vi "R45_1-RT.vi"() -> ()   [LabVIEW 2016]
uses:
  <vilib>/rvi/interface/nirviOpenFPGA/nirviOpenFPGA.xnode
  <vilib>/rvi/interface/nirviReadWriteControl/nirviReadWriteControl.xnode
  Common-Control/Beamline sections/R45/R45_1/R45_1-FPGA.vi
  <vilib>/rvi/errors/niLvFpgaAdjustHostInterfaceError.vi
  <vilib>/Utility/error.llb/Error Cluster From Error Code.vi
  NiFpgaLv.dll
  Glassman Control.ctl
  GP307 cluster.ctl
  Controls/GV states.ctl
  Controls/Faraday cup states.ctl
  Controls/Aperture states.ctl
  Cryo Readback.ctl
  <vilib>/NI_Real-Time Target Support.lvlib
  FPGA Bitfiles/PRIMEControl2017_FPGATarget10_R45-1-FPGA_JlC5-fMslM8.lvbitx
  <vilib>/FPGAPlugInAG/cRIO-9067/niLvFpga_Open_cRIO-9067.vi
panel:
  in  "Tab Control":T1(tab)
  out "Left-Steerer voltage set":dbl
  out "Left-Steerer HV Enable":bool
  out "Right-Steerer HV Enable":bool
  out "Right-Steerer voltage set":dbl
  out "Up-Steerer Voltage Set":dbl
  out "Up-Steerer HV Enable":bool
  out "Down-Steerer HV Enable":bool
  out "Down-Steerer Voltage Set":dbl
  out "Up Steerer readback.I-monitor":fxp<+/-,26,5>
  out "Up Steerer readback.V-monitor":fxp<+/-,26,7>
  out "Down Steerer readback.I-monitor":fxp<+/-,26,5>
  out "Down Steerer readback.V-monitor":fxp<+/-,26,7>
  out "Left Steerer readback.I-monitor":fxp<+/-,26,5>
  out "Left Steerer readback.V-monitor":fxp<+/-,26,7>
  out "Right Steerer readback.I-monitor":fxp<+/-,26,5>
  out "Right Steerer readback.V-monitor":fxp<+/-,26,7>
  out "Cryo status":u8[](array[numeric])
  out "Cryo On-time":u8[](array[numeric])
  out "Cryo 1st stage temp":u8[](array[numeric])
  out "2nd stage temp":u8[](array[numeric])
  out "Time since repurge":u8[](array[numeric])
  out "Vac cluster 2 Interlock":bool
  out "Vac cluster 2 Interlock bypass":bool
  out "Vac cluster 1 interlock bypass":bool
  out "Status":string
  out "On-time":string
  out "1st Stage Temp":string
  out "2nd Stage Temp":string
  out "Time since re-purge":string
  out "Cryo Readback":T2
  out "Vac Cluster 1 Ion Gauge 1":u8[](array[numeric])
  out "Vac Cluster 1 Convectron 1":u8[](array[numeric])
  out "Switch Image Convectron 1":dbl
  out "Switch Image Vac Cluster":T3
  out "Switch Image Ion Gauge 1":dbl
  out "Vac Cluster 1 Ion Gauge 2":u8[](array[numeric])
  out "Vac Cluster 1 Convectron 2":u8[](array[numeric])
  out "Cryo Pump GV status 2":T4
  out "Cryo Pump GV status":T5
  out "Beamline GV 1 status 2":T4
  out "Beamline GV 1 status":T5
  out "Switch Image FC Position":cluster{"IN sensor":bool, "OUT sensor":bool}
  out "Switch Image Aperture Position":cluster{"IN sensor":bool, "OUT sensor":bool}
  out "Aperture Status":T6
  out "FC Status":T7
  out "Cryo Pump GV Actuator":bool
  out "Switch Mag Aperture actuator":bool
  out "Switch Mag FC actuator":bool
  out "Beamline GV 1 Actuator":bool
  out "Error Reporter":errorcluster
  out "Interlock loop error":errorcluster
  out "Actuator-Sensor Loop error":errorcluster
  out "Cryo loop error":errorcluster
  out "Vac cluster loop error":errorcluster
  out "HV readback loop error":errorcluster
  out "HV control loop error":errorcluster
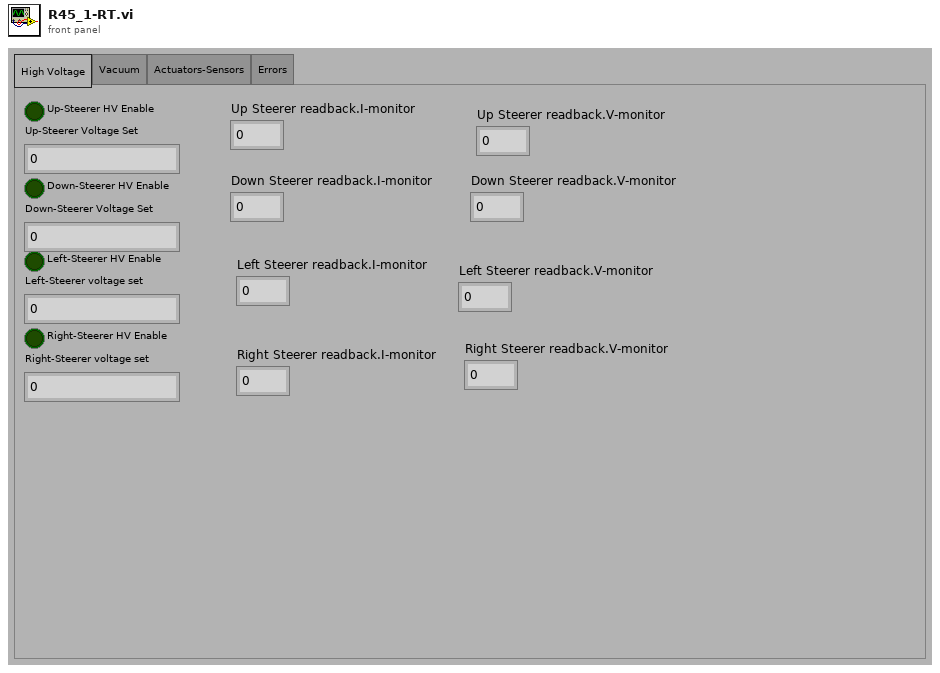
[diagram p1: front panel]
types:
  T1 = enum32{"High Voltage", "Vacuum", "Actuators-Sensors", "Errors"}
  T2 = typedef "Cryo Readback.ctl" = cluster{"Status":string, "On-time":string, "1st Stage Temp":string, "2nd Stage Temp":string, "Time since re-purge":string}
  T3 = typedef "GP307 cluster.ctl" = cluster{"Ion gauge 1":string, "Convectron  Gauge 1 ":string, "Ion Gauge 2":string, "Convectrom Gauge 2":string}
  T4 = cluster{"OPEN sensor":bool, "Closed sensor":bool}
  T5 = typedef "GV states.ctl" = enum16{"status unclear", "closed", "open"}
  T6 = typedef "Aperture states.ctl" = enum16{"Aperture status unclear", "Aperture in", "Aperture out"}
  T7 = typedef "Faraday cup states.ctl" = enum16{"FC status unclear", "FC in", "FC out"}
  T8 = typedef "Glassman Control.ctl" = cluster{"V-program":fxp<+/-,16,5>, "HV Enable":bool}
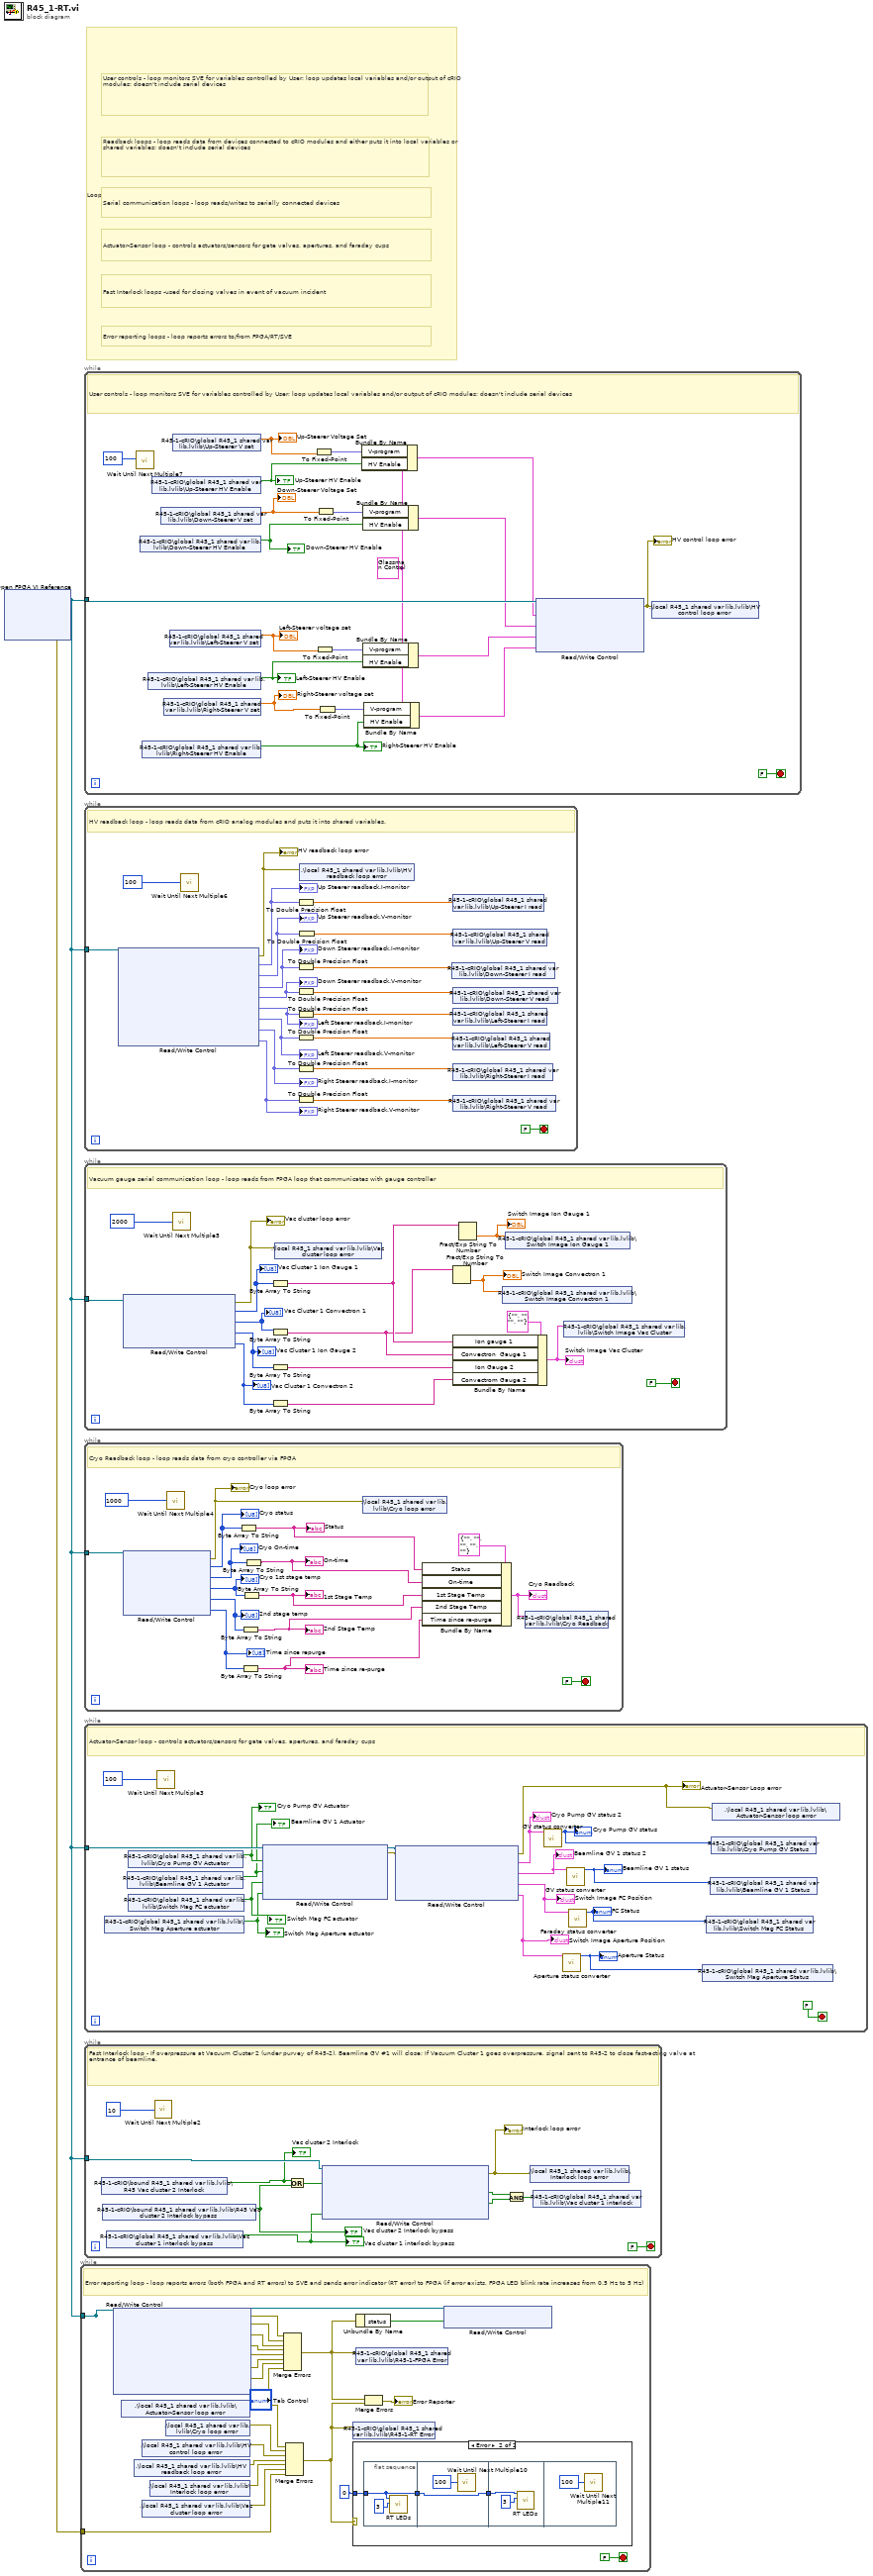
[diagram p0: block diagram]
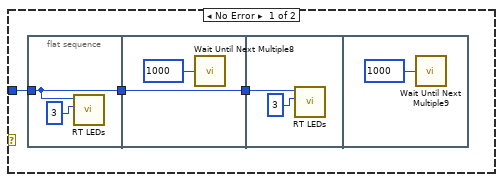
[diagram p2: hidden frame]
diagram:
  # "Actuator-Sensor loop - controls actuators/sensors for gate valves, apertures, and faraday cups"
  # "Fast Interlock loops -used for closing valves in event of vacuum incident"
  # "Error reporting loops - loop reports errors to/from FPGA/RT/SVE"
  # "Serial communication loops - loop reads/writes to serially connected devices"
  # "Readback loops - loop reads data from devices connected to cRIO modules and either puts it into local variables or shared variables; doesn't include serial devices"
  # "User controls - loop monitors SVE for variables controlled by User; loop updates local variables and/or output of cRIO modules; doesn't include serial devices"
  # "Loop legend - loops are color coded by responsibility"
  n1 = xnode "Open FPGA VI Reference"() -> ("FPGA VI Reference Out"=w2:refnum<k20>, "error out"=w1:errorcluster)  [unwired: 2 in]
  n2 = while {
    tunnel: [w25] -> _
    tunnel: w2 -> [w25]
    tunnel: w1 -> [w5]
    stop <- FALSE stop-if-true
    # "Error reporting loop - loop reports errors (both FPGA and RT errors) to SVE and sends error indicator (RT error) to FPGA (if error exists, FPGA LED blink rate increases from 0.5 Hz to 5 Hz)"
    n3 = xnode "Read/Write Control"("FPGA VI Reference In"=w25) -> ("FPGA VI Reference Out"=w15:refnum<k20>, "error out"=w24:errorcluster, "Vac and GV interlock error"=w23:errorcluster, "Position-Sensor readback error"=w22:errorcluster, "Cup-Aperture Control Loop Error"=w21:errorcluster, "Cryo pump error"=w20:errorcluster, "HV readback error"=w19:errorcluster, "HV Control error"=w18:errorcluster, "Vacuum Gauge 1 error"=w17:errorcluster)  [unwired: 1 in]
    n4 = shared-variable ".\\local R45_1 shared var lib.lvlib\\Actuator-Sensor loop error"() -> (w11:errorcluster)  [unwired: 1 in, 1 out]
    n5 = shared-variable ".\\local R45_1 shared var lib.lvlib\\HV readback loop error"() -> (w8:errorcluster)  [unwired: 1 in, 1 out]
    n6 = shared-variable ".\\local R45_1 shared var lib.lvlib\\HV control loop error"() -> (w9:errorcluster)  [unwired: 1 in, 1 out]
    n7 = shared-variable ".\\local R45_1 shared var lib.lvlib\\Vac cluster loop error"() -> (w6:errorcluster)  [unwired: 1 in, 1 out]
    n8 = shared-variable ".\\local R45_1 shared var lib.lvlib\\Interlock loop error"() -> (w7:errorcluster)  [unwired: 1 in, 1 out]
    n9 = shared-variable ".\\local R45_1 shared var lib.lvlib\\Cryo loop error"() -> (w10:errorcluster)  [unwired: 1 in, 1 out]
    n10 = Merge Errors(w24, w23, w22, w21, w20, w19, w18, w17) -> (w16:errorcluster)
    n11 = Merge Errors(w11, w10, w9, w8, w7, w6, w5) -> (w3:errorcluster)
    n12 = case shown="Error" w3 {
      tunnel: 0 -> [w28 w36]
      frame No Error {
        n13 = flat-sequence {
          tunnel: w28 -> [w29]
          tunnel: [w29] -> w26
          tunnel: [w31] -> w27
          tunnel: w26 -> [w31]
          tunnel: w27 -> [w33]
          frame #0 {
            n14 = call <vilib>:"RT LEDs.vi"("State"=3, "LED Num"=w29) -> ()  [unwired: 4 in, 2 out]
          }
          frame #1 {
            n15 = call "Wait Until Next Multiple8"("Count(mSec)"=u16 1000) -> ()  [unwired: 1 out]
          }
          frame #2 {
            n16 = call <vilib>:"RT LEDs.vi"("State"=3, "LED Num"=w33) -> ()  [unwired: 4 in, 2 out]
          }
          frame #3 {
            n17 = call "Wait Until Next Multiple9"("Count(mSec)"=u16 1000) -> ()  [unwired: 1 out]
          }
        }
      }
      frame Error {
        n18 = flat-sequence {
          tunnel: [w39] -> w38
          tunnel: w36 -> [w39]
          tunnel: w38 -> [w41]
          tunnel: [w41] -> w37
          tunnel: w37 -> [w43]
          frame #0 {
            n19 = call <vilib>:"RT LEDs.vi"("State"=3, "LED Num"=w39) -> ()  [unwired: 4 in, 2 out]
          }
          frame #1 {
            n20 = call "Wait Until Next Multiple10"("Count(mSec)"=u16 100) -> ()  [unwired: 1 out]
          }
          frame #2 {
            n21 = call <vilib>:"RT LEDs.vi"("State"=3, "LED Num"=w43) -> ()  [unwired: 4 in, 2 out]
          }
          frame #3 {
            n22 = call "Wait Until Next Multiple11"("Count(mSec)"=u16 100) -> ()  [unwired: 1 out]
          }
        }
      }
    }
    n23 = shared-variable "R45-1-cRIO\\global R45_1 shared var lib.lvlib\\R45-1-RT Error"(w3) -> ()  [unwired: 1 in, 1 out]
    n24 = shared-variable "R45-1-cRIO\\global R45_1 shared var lib.lvlib\\R45-1-FPGA Error"(w16) -> ()  [unwired: 1 in, 1 out]
    n25 = Unbundle By Name(w16) -> ("status"=w14:bool)
    n26 = Merge Errors(w16, w3) -> (→"Error Reporter":errorcluster)
    n27 = xnode "Read/Write Control"("FPGA VI Reference In"=w15, "RT error"=w14) -> ()  [unwired: 1 in, 2 out]
  }
  n28 = while {
    tunnel: w2 -> [w66]
    stop <- FALSE stop-if-true
    w55 = T8 {"V-program"=0.0, "HV Enable"=FALSE} ("Glassman Control")
    # "User controls - loop monitors SVE for variables controlled by User; loop updates local variables and/or output of cRIO modules; doesn't include serial devices"
    n29 = call "Wait Until Next Multiple7"("Count(mSec)"=u32 100 ("millisecond multiple")) -> ()  [unwired: 1 out]
    n30 = shared-variable "R45-1-cRIO\\global R45_1 shared var lib.lvlib\\Down-Steerer HV Enable"() -> (w51:bool)  [unwired: 1 in, 1 out]
    "Down-Steerer HV Enable" <- w51
    n31 = shared-variable "R45-1-cRIO\\global R45_1 shared var lib.lvlib\\Right-Steerer HV Enable"() -> (w47:bool)  [unwired: 1 in, 1 out]
    "Right-Steerer HV Enable" <- w47
    n32 = shared-variable "R45-1-cRIO\\global R45_1 shared var lib.lvlib\\Left-Steerer HV Enable"() -> (w49:bool)  [unwired: 1 in, 1 out]
    "Left-Steerer HV Enable" <- w49
    n33 = shared-variable "R45-1-cRIO\\global R45_1 shared var lib.lvlib\\Up-Steerer HV Enable"() -> (w54:bool)  [unwired: 1 in, 1 out]
    "Up-Steerer HV Enable" <- w54
    n34 = shared-variable "R45-1-cRIO\\global R45_1 shared var lib.lvlib\\Down-Steerer V set"() -> (w52:dbl)  [unwired: 1 in, 1 out]
    "Down-Steerer Voltage Set" <- w52
    n35 = shared-variable "R45-1-cRIO\\global R45_1 shared var lib.lvlib\\Right-Steerer V set"() -> (w48:dbl)  [unwired: 1 in, 1 out]
    "Right-Steerer voltage set" <- w48
    n36 = shared-variable "R45-1-cRIO\\global R45_1 shared var lib.lvlib\\Left-Steerer V set"() -> (w50:dbl)  [unwired: 1 in, 1 out]
    "Left-Steerer voltage set" <- w50
    n37 = shared-variable "R45-1-cRIO\\global R45_1 shared var lib.lvlib\\Up-Steerer V set"() -> (w53:dbl)  [unwired: 1 in, 1 out]
    "Up-Steerer Voltage Set" <- w53
    n38 = To Fixed-Point(number=w53) -> (fixed-point=w59:fxp<+/-,20,5>)  [unwired: 1 in]
    n39 = To Fixed-Point(number=w50) -> (fixed-point=w63:fxp<+/-,20,5>)  [unwired: 1 in]
    n40 = To Fixed-Point(number=w52) -> (fixed-point=w58:fxp<+/-,20,5>)  [unwired: 1 in]
    n41 = To Fixed-Point(number=w48) -> (fixed-point=w62:fxp<+/-,20,5>)  [unwired: 1 in]
    n42 = Bundle By Name(cluster=w55, "V-program"=w59, "HV Enable"=w54) -> (w56:T8)
    n43 = Bundle By Name(cluster=w55, "V-program"=w58, "HV Enable"=w51) -> (w57:T8)
    n44 = Bundle By Name(cluster=w55, "V-program"=w63, "HV Enable"=w49) -> (w60:T8)
    n45 = Bundle By Name(cluster=w55, "V-program"=w62, "HV Enable"=w47) -> (w61:T8)
    n46 = xnode "Read/Write Control"("FPGA VI Reference In"=w66, "Up Steerer Voltage set"=w56, "Down Steerer Voltage set"=w57, "Left Steerer Voltage set"=w60, "Right Steerer Voltage set"=w61) -> ("error out"=w64:errorcluster)  [unwired: 1 in, 1 out]
    "HV control loop error" <- w64
    n47 = shared-variable ".\\local R45_1 shared var lib.lvlib\\HV control loop error"(w64) -> ()  [unwired: 1 in, 1 out]
  }
  n48 = while {
    tunnel: w2 -> [w86]
    stop <- FALSE stop-if-true
    # "HV readback loop - loop reads data from cRIO analog modules and puts it into shared variables."
    n49 = xnode "Read/Write Control"("FPGA VI Reference In"=w86) -> ("error out"=w84:errorcluster, "Up Steerer readback.I-monitor"=w83:fxp<+/-,16,5>, "Up Steerer readback.V-monitor"=w82:fxp<+/-,16,5>, "Down Steerer readback.I-monitor"=w81:fxp<+/-,16,5>, "Down Steerer readback.V-monitor"=w80:fxp<+/-,16,5>, "Left Steerer readback.I-monitor"=w79:fxp<+/-,16,5>, "Left Steerer readback.V-monitor"=w78:fxp<+/-,16,5>, "Right Steerer readback.I-monitor"=w77:fxp<+/-,16,5>, "Right Steerer readback.V-monitor"=w76:fxp<+/-,16,5>)  [unwired: 1 in, 1 out]
    "Up Steerer readback.I-monitor" <- w83
    "Up Steerer readback.V-monitor" <- w82
    "Down Steerer readback.I-monitor" <- w81
    "Down Steerer readback.V-monitor" <- w80
    "Left Steerer readback.I-monitor" <- w79
    "Left Steerer readback.V-monitor" <- w78
    "Right Steerer readback.I-monitor" <- w77
    "Right Steerer readback.V-monitor" <- w76
    "HV readback loop error" <- w84
    n50 = call "Wait Until Next Multiple6"("Count(mSec)"=u32 100 ("millisecond multiple")) -> ()  [unwired: 1 out]
    n51 = To Double Precision Float(number=w83) -> (double precision float=w75:dbl)
    n52 = To Double Precision Float(number=w81) -> (double precision float=w72:dbl)
    n53 = To Double Precision Float(number=w80) -> (double precision float=w71:dbl)
    n54 = To Double Precision Float(number=w79) -> (double precision float=w70:dbl)
    n55 = To Double Precision Float(number=w78) -> (double precision float=w69:dbl)
    n56 = To Double Precision Float(number=w77) -> (double precision float=w68:dbl)
    n57 = To Double Precision Float(number=w76) -> (double precision float=w74:dbl)
    n58 = To Double Precision Float(number=w82) -> (double precision float=w73:dbl)
    n59 = shared-variable ".\\local R45_1 shared var lib.lvlib\\HV readback loop error"(w84) -> ()  [unwired: 1 in, 1 out]
    n60 = shared-variable "R45-1-cRIO\\global R45_1 shared var lib.lvlib\\Down-Steerer I read"(w72) -> ()  [unwired: 1 in, 1 out]
    n61 = shared-variable "R45-1-cRIO\\global R45_1 shared var lib.lvlib\\Up-Steerer I read"(w75) -> ()  [unwired: 1 in, 1 out]
    n62 = shared-variable "R45-1-cRIO\\global R45_1 shared var lib.lvlib\\Down-Steerer V read"(w71) -> ()  [unwired: 1 in, 1 out]
    n63 = shared-variable "R45-1-cRIO\\global R45_1 shared var lib.lvlib\\Left-Steerer I read"(w70) -> ()  [unwired: 1 in, 1 out]
    n64 = shared-variable "R45-1-cRIO\\global R45_1 shared var lib.lvlib\\Left-Steerer V read"(w69) -> ()  [unwired: 1 in, 1 out]
    n65 = shared-variable "R45-1-cRIO\\global R45_1 shared var lib.lvlib\\Right-Steerer I read"(w68) -> ()  [unwired: 1 in, 1 out]
    n66 = shared-variable "R45-1-cRIO\\global R45_1 shared var lib.lvlib\\Right-Steerer V read"(w74) -> ()  [unwired: 1 in, 1 out]
    n67 = shared-variable "R45-1-cRIO\\global R45_1 shared var lib.lvlib\\Up-Steerer V read"(w73) -> ()  [unwired: 1 in, 1 out]
  }
  n68 = while {
    tunnel: w2 -> [w97]
    stop <- FALSE stop-if-true
    # "Vacuum gauge serial communication loop - loop reads from FPGA loop that communicates with gauge controller"
    n69 = xnode "Read/Write Control"("FPGA VI Reference In"=w97) -> ("error out"=w90:errorcluster, "Vac Cluster 1 Ion Gauge 1"=w98:u8[], "Vac Cluster 1 Convectron 1"=w93:u8[], "Vac Cluster 1 Ion Gauge 2"=w99:u8[], "Vac Cluster 1 Convectron 2"=w100:u8[])  [unwired: 1 in, 1 out]
    "Vac Cluster 1 Ion Gauge 1" <- w98
    "Vac Cluster 1 Convectron 1" <- w93
    "Vac Cluster 1 Ion Gauge 2" <- w99
    "Vac Cluster 1 Convectron 2" <- w100
    "Vac cluster loop error" <- w90
    n70 = call "Wait Until Next Multiple5"("Count(mSec)"=u32 2000 ("millisecond multiple")) -> ()  [unwired: 1 out]
    n71 = Byte Array To String(unsigned byte array=w98) -> (string=w94:string)
    n72 = Byte Array To String(unsigned byte array=w93) -> (string=w92:string)
    n73 = Byte Array To String(unsigned byte array=w99) -> (string=w101:string)
    n74 = Byte Array To String(unsigned byte array=w100) -> (string=w102:string)
    n75 = shared-variable ".\\local R45_1 shared var lib.lvlib\\Vac cluster loop error"(w90) -> ()  [unwired: 1 in, 1 out]
    n76 = Bundle By Name(cluster=T3 {"Ion gauge 1"="", "Convectron  Gauge 1 "="", "Ion Gauge 2"="", "Convectrom Gauge 2"=""} ("Ion gauge cluster control"), "Ion gauge 1"=w94, "Convectron  Gauge 1"=w92, "Ion Gauge 2"=w101, "Convectrom Gauge 2"=w102) -> (w95:T3)
    "Switch Image Vac Cluster" <- w95
    n77 = Fract/Exp String To Number(string=w92) -> (number=w89:dbl)  [unwired: 3 in, 1 out]
    "Switch Image Convectron 1" <- w89
    n78 = Fract/Exp String To Number(string=w94) -> (number=w91:dbl)  [unwired: 3 in, 1 out]
    "Switch Image Ion Gauge 1" <- w91
    n79 = shared-variable "R45-1-cRIO\\global R45_1 shared var lib.lvlib\\Switch Image Convectron 1"(w89) -> ()  [unwired: 1 in, 1 out]
    n80 = shared-variable "R45-1-cRIO\\global R45_1 shared var lib.lvlib\\Switch Image Ion Gauge 1"(w91) -> ()  [unwired: 1 in, 1 out]
    n81 = shared-variable "R45-1-cRIO\\global R45_1 shared var lib.lvlib\\Switch Image Vac Cluster"(w95) -> ()  [unwired: 1 in, 1 out]
  }
  n82 = while {
    tunnel: w2 -> [w117]
    stop <- FALSE stop-if-true
    # "Cryo Readback loop - loop reads data from cryo controller via FPGA"
    n83 = xnode "Read/Write Control"("FPGA VI Reference In"=w117) -> ("error out"=w113:errorcluster, "Cryo status"=w114:u8[], "Cryo On-time"=w115:u8[], "Cryo 1st stage temp"=w116:u8[], "2nd stage temp"=w112:u8[], "Time since repurge"=w111:u8[])  [unwired: 1 in, 1 out]
    "Cryo status" <- w114
    "Cryo On-time" <- w115
    "Cryo 1st stage temp" <- w116
    "Cryo loop error" <- w113
    "2nd stage temp" <- w112
    "Time since repurge" <- w111
    n84 = call "Wait Until Next Multiple4"("Count(mSec)"=u32 1000 ("millisecond multiple")) -> ()  [unwired: 1 out]
    n85 = Byte Array To String(unsigned byte array=w114) -> (string=w105:string)
    "Status" <- w105
    n86 = Byte Array To String(unsigned byte array=w112) -> (string=w104:string)
    "2nd Stage Temp" <- w104
    n87 = Byte Array To String(unsigned byte array=w111) -> (string=w108:string)
    "Time since re-purge" <- w108
    n88 = Byte Array To String(unsigned byte array=w116) -> (string=w107:string)
    "1st Stage Temp" <- w107
    n89 = Byte Array To String(unsigned byte array=w115) -> (string=w106:string)
    "On-time" <- w106
    n90 = shared-variable ".\\local R45_1 shared var lib.lvlib\\Cryo loop error"(w113) -> ()  [unwired: 1 in, 1 out]
    n91 = Bundle By Name(cluster=T2 {"Status"="", "On-time"="", "1st Stage Temp"="", "2nd Stage Temp"="", "Time since re-purge"=""} ("Cryo Readback"), "Status"=w105, "On-time"=w106, "1st Stage Temp"=w107, "2nd Stage Temp"=w104, "Time since re-purge"=w108) -> (w103:T2)
    "Cryo Readback" <- w103
    n92 = shared-variable "R45-1-cRIO\\global R45_1 shared var lib.lvlib\\Cryo Readback"(w103) -> ()  [unwired: 1 in, 1 out]
  }
  n93 = while {
    tunnel: w2 -> [w136]
    stop <- FALSE stop-if-true
    # "Actuator-Sensor loop - controls actuators/sensors for gate valves, apertures, and faraday cups"
    n94 = shared-variable "R45-1-cRIO\\global R45_1 shared var lib.lvlib\\Switch Mag Aperture actuator"() -> (w120:bool)  [unwired: 1 in, 1 out]
    "Switch Mag Aperture actuator" <- w120
    n95 = shared-variable "R45-1-cRIO\\global R45_1 shared var lib.lvlib\\Beamline GV 1 Actuator"() -> (w122:bool)  [unwired: 1 in, 1 out]
    "Beamline GV 1 Actuator" <- w122
    n96 = shared-variable "R45-1-cRIO\\global R45_1 shared var lib.lvlib\\Cryo Pump GV Actuator"() -> (w123:bool)  [unwired: 1 in, 1 out]
    "Cryo Pump GV Actuator" <- w123
    n97 = shared-variable "R45-1-cRIO\\global R45_1 shared var lib.lvlib\\Switch Mag FC actuator"() -> (w121:bool)  [unwired: 1 in, 1 out]
    "Switch Mag FC actuator" <- w121
    n98 = call "Wait Until Next Multiple3"("Count(mSec)"=u32 100 ("millisecond multiple")) -> ()  [unwired: 1 out]
    n99 = xnode "Read/Write Control"("FPGA VI Reference In"=w136, "Cryo GV actuator"=w123, "Beamline GV 1 actuator"=w122, "Switch Mag FC actuator"=w121, "Switch Mag Aperture actuator"=w120) -> ("FPGA VI Reference Out"=w134:refnum<k20>, "error out"=w133:errorcluster)  [unwired: 1 in]
    n100 = xnode "Read/Write Control"("FPGA VI Reference In"=w134, "error in"=w133) -> ("error out"=w124:errorcluster, "Cryo Pump GV position"=w131:T4, "Beamline GV 1 position"=w129:T4, "Switch Mag FC Position"=w128:cluster{"IN sensor":bool, "OUT sensor":bool}, "Switch Mag Aperture Position"=w127:cluster{"IN sensor":bool, "OUT sensor":bool})  [unwired: 1 out]
    "Cryo Pump GV status 2" <- w131
    "Beamline GV 1 status 2" <- w129
    "Switch Image FC Position" <- w128
    "Switch Image Aperture Position" <- w127
    "Actuator-Sensor Loop error" <- w124
    n101 = call "GV status converter.vi"("Gate Valve"=w131) -> ("GV Status"=w132:T5)  [unwired: 10 in]
    "Cryo Pump GV status" <- w132
    n102 = call "Aperture status converter.vi"("Aperture Position"=w127) -> ("Aperture Status"=w126:T6)  [unwired: 10 in]
    "Aperture Status" <- w126
    n103 = call "GV status converter.vi"("Gate Valve"=w129) -> ("GV Status"=w130:T5)  [unwired: 10 in]
    "Beamline GV 1 status" <- w130
    n104 = call "Faraday status converter.vi"("FC Position"=w128) -> ("FC Status"=w125:T7)  [unwired: 10 in]
    "FC Status" <- w125
    n105 = shared-variable "R45-1-cRIO\\global R45_1 shared var lib.lvlib\\Switch Mag Aperture Status"(w126) -> ()  [unwired: 1 in, 1 out]
    n106 = shared-variable "R45-1-cRIO\\global R45_1 shared var lib.lvlib\\Switch Mag FC Status"(w125) -> ()  [unwired: 1 in, 1 out]
    n107 = shared-variable "R45-1-cRIO\\global R45_1 shared var lib.lvlib\\Beamline GV 1 Status"(w130) -> ()  [unwired: 1 in, 1 out]
    n108 = shared-variable "R45-1-cRIO\\global R45_1 shared var lib.lvlib\\Cryo Pump GV Status"(w132) -> ()  [unwired: 1 in, 1 out]
    n109 = shared-variable ".\\local R45_1 shared var lib.lvlib\\Actuator-Sensor loop error"(w124) -> ()  [unwired: 1 in, 1 out]
  }
  n110 = while {
    tunnel: w2 -> [w144]
    stop <- FALSE stop-if-true
    # "Fast Interlock loop - If overpressure at Vacuum Cluster 2 (under purvey of R45-2), Beamline GV #1 will close; If Vacuum Cluster 1 goes overpressure, signal sent to R45-2 to close fast-acting valve at entrance of beamline."
    n111 = shared-variable "R45-1-cRIO\\bound R45_1 shared var lib.lvlib\\R45 Vac cluster 2 Interlock"() -> (w140:bool)  [unwired: 1 in, 1 out]
    "Vac cluster 2 Interlock" <- w140
    n112 = shared-variable "R45-1-cRIO\\bound R45_1 shared var lib.lvlib\\R45 Vac cluster 2 Interlock bypass"() -> (w139:bool)  [unwired: 1 in, 1 out]
    "Vac cluster 2 Interlock bypass" <- w139
    n113 = shared-variable "R45-1-cRIO\\global R45_1 shared var lib.lvlib\\Vac cluster 1 interlock bypass"() -> (w138:bool)  [unwired: 1 in, 1 out]
    "Vac cluster 1 interlock bypass" <- w138
    n114 = call "Wait Until Next Multiple2"("Count(mSec)"=u32 10 ("millisecond multiple")) -> ()  [unwired: 1 out]
    n115 = Or(x=w140, y=w139) -> (x .or. y?=w141:bool)
    n116 = xnode "Read/Write Control"("FPGA VI Reference In"=w144, "Vac cluster 2 Ion Gauge Interlock"=w141, "Vac Cluster 1 Interlock bypass"=w138) -> ("error out"=w143:errorcluster, "Vac cluster 1 Ion Gauge Interlock"=w147:bool, "Vac cluster 1 Convectron Gauge Interlock"=w146:bool)  [unwired: 1 in, 1 out]
    "Interlock loop error" <- w143
    n117 = And(x=w147, y=w146) -> (x .and. y?=w145:bool)
    n118 = shared-variable ".\\local R45_1 shared var lib.lvlib\\Interlock loop error"(w143) -> ()  [unwired: 1 in, 1 out]
    n119 = shared-variable "R45-1-cRIO\\global R45_1 shared var lib.lvlib\\Vac cluster 1 interlock"(w145) -> ()  [unwired: 1 in, 1 out]
  }
